vi "Control_stage_2.vi"(11 "Stage control":T3={"Up"=FALSE, "Left"=FALSE, "Right"=FALSE, "Down"=FALSE, "Z Down"=FALSE, "Z Up"=FALSE, "X Step Size(um)"=0.0, "Z step size (um)"=0.0, "Y Step Size(um)"=0.0, "Enable x-axis"=TRUE, "Enable y-axis"=TRUE, "Enable z-axis"=TRUE, "Same step size"=FALSE, "Global step size"=10.0, "stop"=FALSE, "Destination"={"X Position"=0.0, "Y Position"=0.0, "Z Position"=0.0}, "Move to destination"=FALSE}) -> (10 "Stage position":T2)   [LabVIEW 2020]
uses:
  typedefs/typedef_stage_control.ctl
  typedefs/typedef_stage_position.ctl
  typedefs/typedef_Z_stack.ctl
panel:
  in  "Z-stack":T1 {"Progress" scale=0.0..100.0}
  out "Error out":errorcluster
  out "Connected":bool=TRUE
  out "FirmwareVersion":string="3.03\r"
  in  "SPIIPLUSCOM660Lib.IAsyncChannel":refnum<k7>
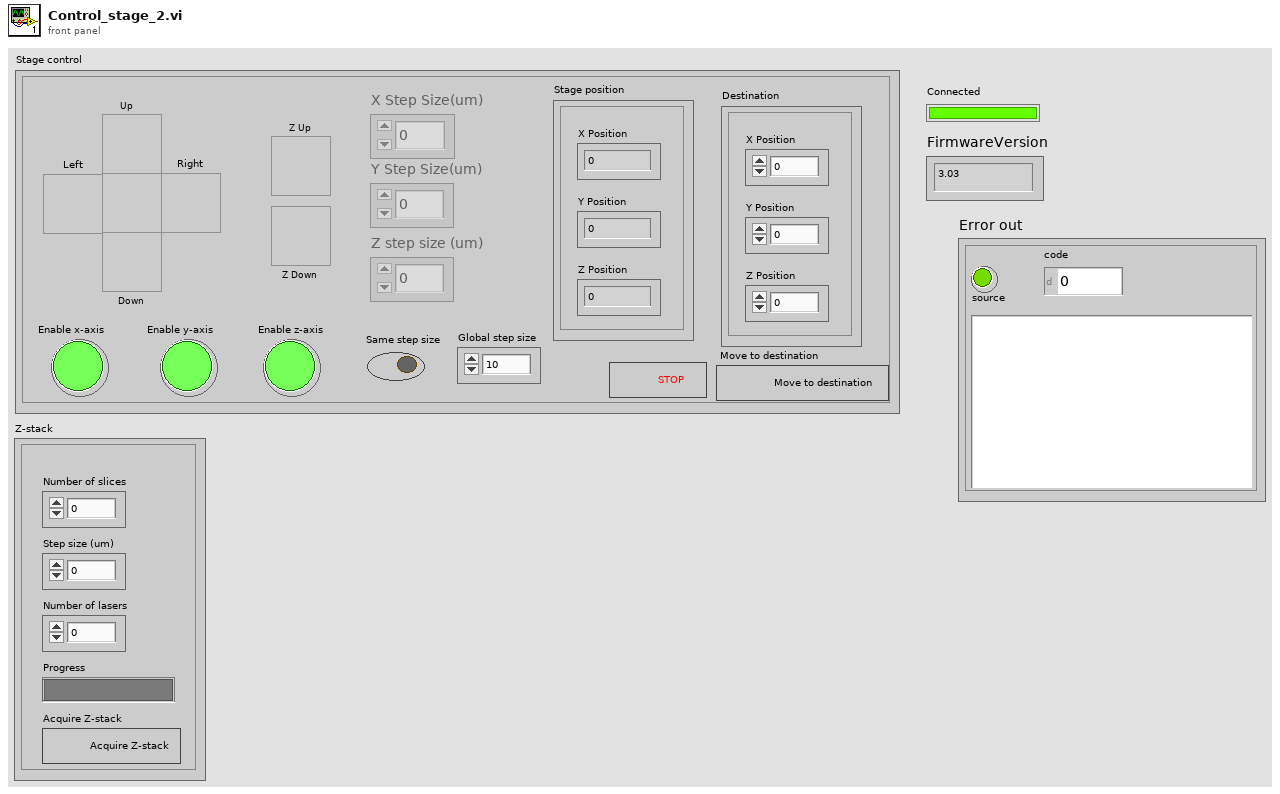
[diagram p1: front panel]
types:
  T1 = typedef "typedef_Z_stack.ctl" = cluster{"Acquire Z-stack":bool, "Step size (um)":dbl, "Number of slices":dbl, "Number of lasers":dbl, "Progress":u8}
  T2 = typedef "typedef_stage_position.ctl" = cluster{"X Position":dbl, "Y Position":dbl, "Z Position":dbl}
  T3 = typedef "typedef_stage_control.ctl" = cluster{"Up":bool, "Left":bool, "Right":bool, "Down":bool, "Z Down":bool, "Z Up":bool, "X Step Size(um)":dbl, "Z step size (um)":dbl, "Y Step Size(um)":dbl, "Enable x-axis":bool, "Enable y-axis":bool, "Enable z-axis":bool, "Same step size":bool, "Global step size":dbl, "stop":bool, "Destination":T2, "Move to destination":bool}
  T4 = enum16{"Initialize", "Verify connection", "Running", "Closing"}
  T5 = enum8{"Enabled", "Disabled", "Disabled and Grayed Out"}
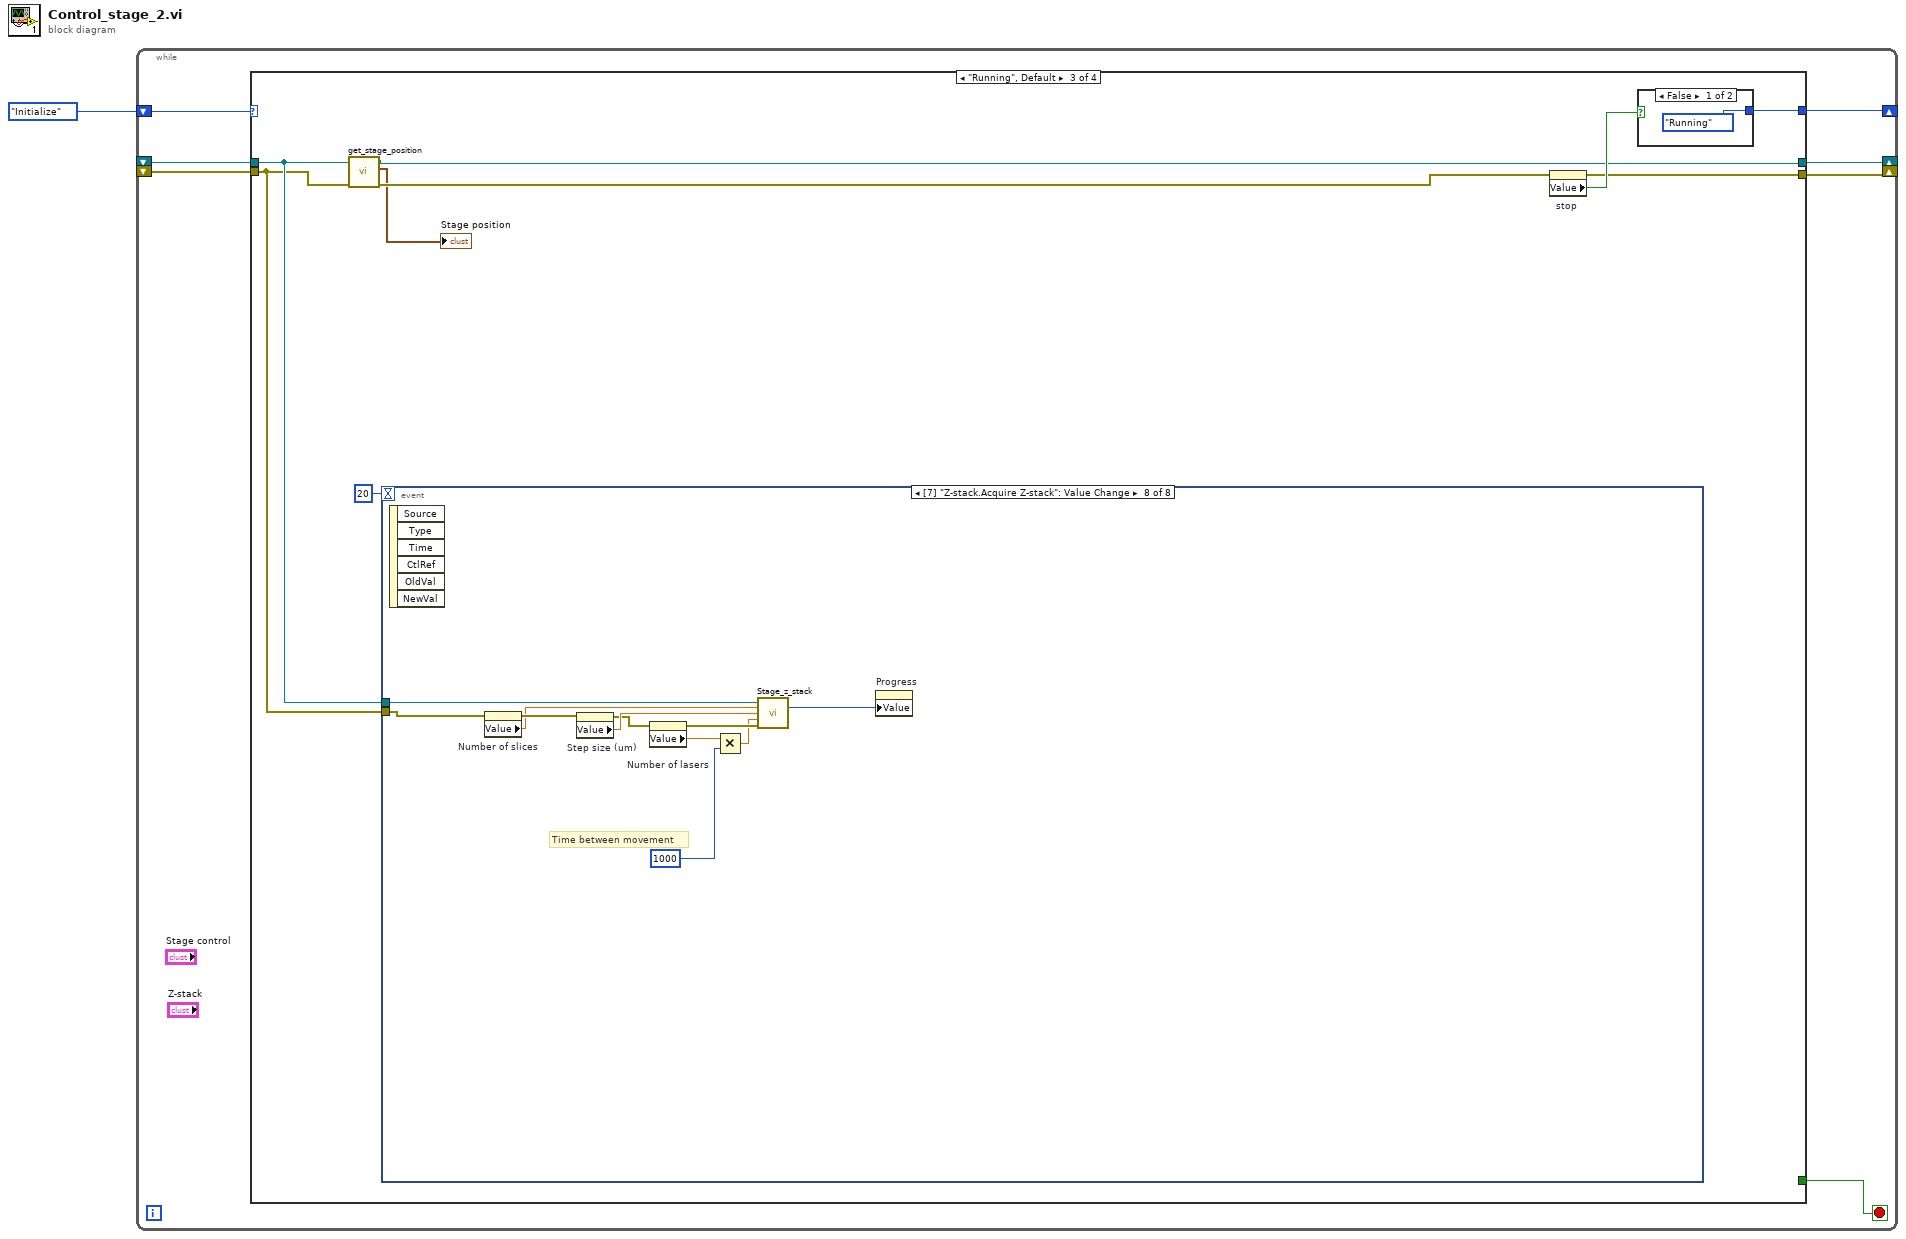
[diagram p0: block diagram]
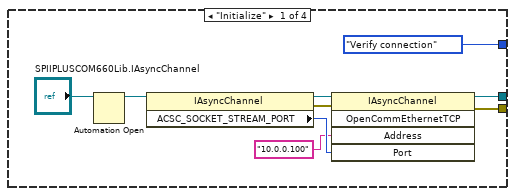
[diagram p2: hidden frame]
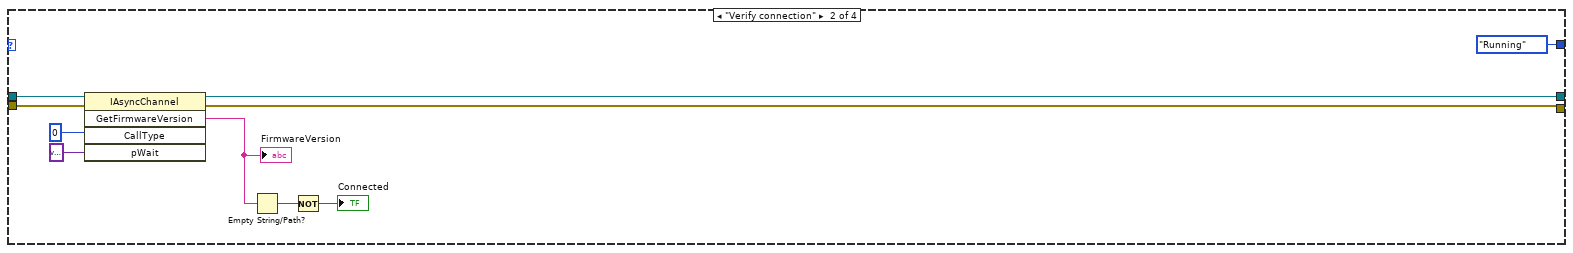
[diagram p3: hidden frame]
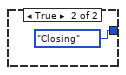
[diagram p4: hidden frame]
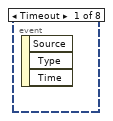
[diagram p5: hidden frame]
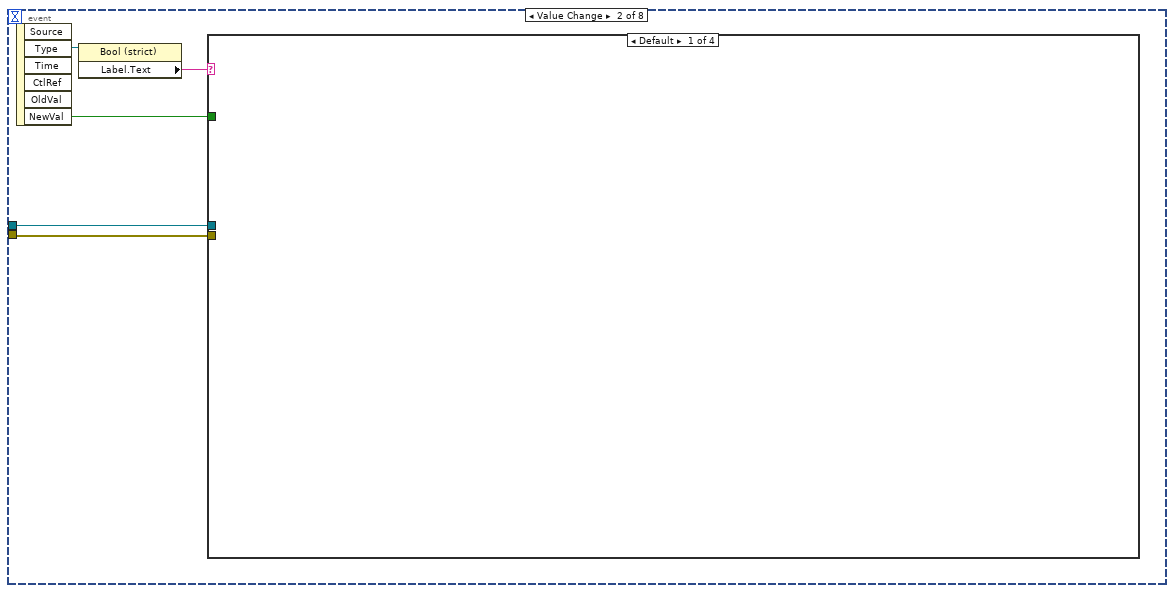
[diagram p6: hidden frame]
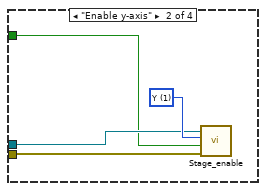
[diagram p7: hidden frame]
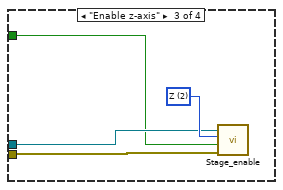
[diagram p8: hidden frame]
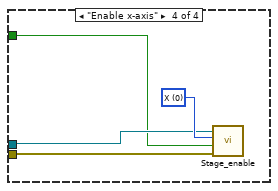
[diagram p9: hidden frame]
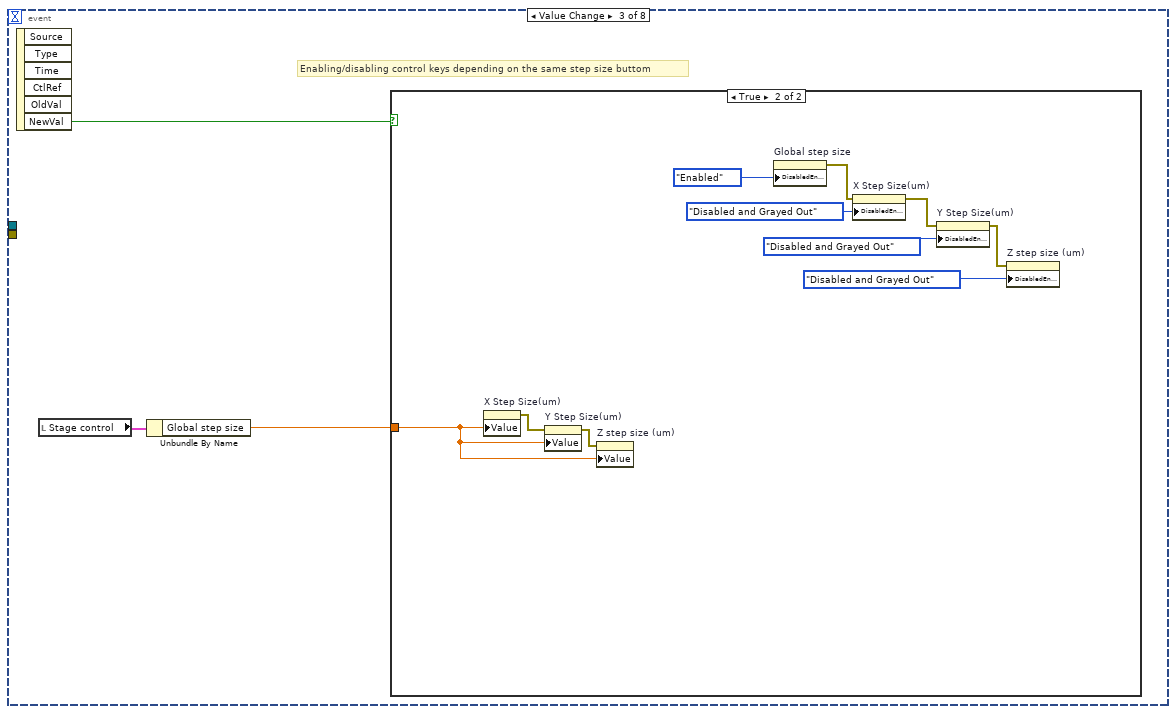
[diagram p10: hidden frame]
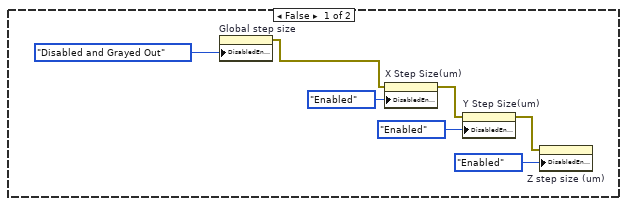
[diagram p11: hidden frame]
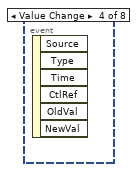
[diagram p12: hidden frame]
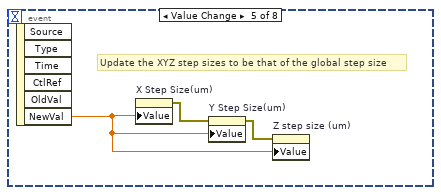
[diagram p13: hidden frame]
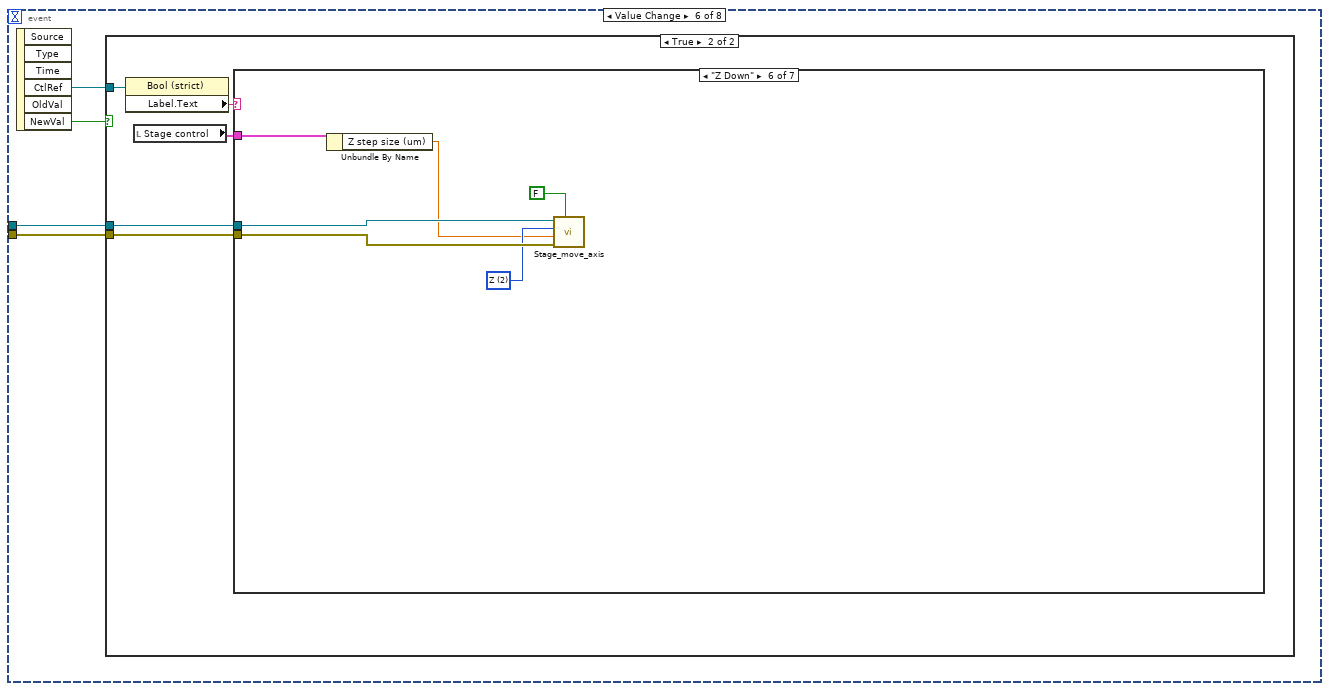
[diagram p14: hidden frame]
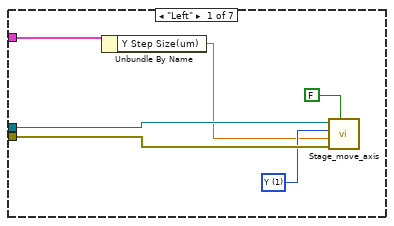
[diagram p16: hidden frame]
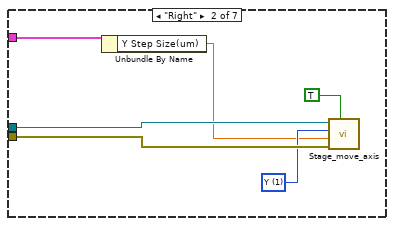
[diagram p17: hidden frame]
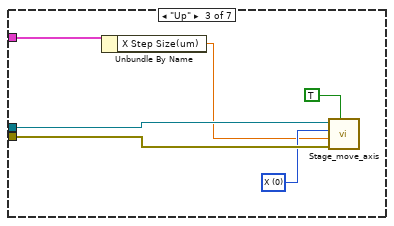
[diagram p18: hidden frame]
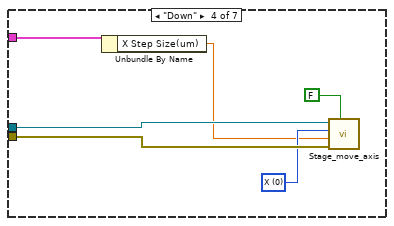
[diagram p19: hidden frame]
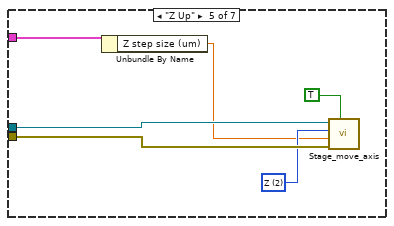
[diagram p20: hidden frame]
diagram:
  n1 = while {
    shift-right: [w4] -> _
    shift-left: T4."Initialize" -> [w7]
    shift-right: [w6] -> _
    shift-left: _ -> [w3]
    shift-right: [w5] -> _
    shift-left: _ -> [w2]
    stop <- w8 stop-if-true
    n2 = case shown="\"Running\", Default" w7 {
      tunnel: [_ _ _ TRUE ("NewVal")] -> w8
      tunnel: [w11 w20 w30 _] -> w6
      tunnel: [w10 w19 w34 _] -> w5
      tunnel: [T4."Verify connection" T4."Running" w36 _] -> w4
      tunnel: w3 -> [_ w22 w32 w163]
      tunnel: w2 -> [_ w21 w31 w162]
      frame "Initialize" {
        n3 = Automation Open(Automation Refnum="SPIIPLUSCOM660Lib.IAsyncChannel") -> (Automation Refnum=w17:refnum<k7>)  [unwired: 3 in, 1 out]
        n4 = property class="IAsyncChannel"(reference=w17) -> (reference out=w16:refnum<k7>, error out=w12:errorcluster, "ACSC_SOCKET_STREAM_PORT"=w14:i32)  [unwired: 1 in]
        n5 = invoke class="IAsyncChannel" method="OpenCommEthernetTCP"(reference=w16, error in=w12, "Address"="10.0.0.100", "Port"=w14) -> (reference out=w11:refnum<k7>, error out=w10:errorcluster)  [unwired: 1 in, 3 out]
      }
      frame "Verify connection" {
        n6 = invoke class="IAsyncChannel" method="GetFirmwareVersion"(reference=w22, error in=w21, "CallType"=u64 0, "pWait"=variant) -> (reference out=w20:refnum<k7>, error out=w19:errorcluster, "GetFirmwareVersion"=w25:string)  [unwired: 1 in, 2 out]
        "FirmwareVersion" <- w25
        n7 = Empty String/Path?(string/path=w25) -> (empty?=w24:bool)
        n8 = Not(x=w24) -> (.not. x?=→"Connected":bool)
      }
      frame "Running", Default {
        n9 = call "get_stage_position.vi"("error IN"=w31, "reference IN"=w32) -> ("error OUT"=w29:errorcluster, "Stage position OUT"=→"Stage position":T2, "reference OUT"=w30:refnum<k7>)  [unwired: 7 in]
        n10 = event shown="[7] \"Z-stack.Acquire Z-stack\": Value Change" {
          selector: _ -> [_ _ _ _ _ _ _ _]
          dyn-events: _ -> [_ _ _ _ _ _ _ _]
          timeout: 20 -> [_ _ _ _ _ _ _ _]
          tunnel: w32 -> [_ w40 _ _ _ w80 w149 w160]
          tunnel: w31 -> [_ w39 _ _ _ w79 w148 w159]
          event Timeout {
            n11 = event-data() -> ()  [unwired: 1 in, 3 out]
          }
          event Value Change {
            n12 = event-data() -> ("CtlRef"=w43:refnum<vi>, "NewVal"=w41:bool)  [unwired: 1 in, 4 out]
            n13 = property class="Bool (strict)"(reference=w43) -> ("Label.Text"=w42:string)  [unwired: 1 in, 2 out]
            n14 = case shown="Default" w42 {
              tunnel: w41 -> [_ w44 w48 w52]
              tunnel: w40 -> [_ w45 w50 w54]
              tunnel: w39 -> [_ w46 w49 w53]
              frame Default {
              }
              frame "Enable y-axis" {
                w47 = u16 1 items=["X", "Y", "Z"] ("Axes Select")
                n15 = call "Stage_enable.vi"("error in (no error)"=w46, "Boolean"=w44, "Axes Select"=w47, "reference"=w45) -> ()  [unwired: 6 in, 2 out]
              }
              frame "Enable z-axis" {
                w51 = u16 2 items=["X", "Y", "Z"] ("Axes Select")
                n16 = call "Stage_enable.vi"("error in (no error)"=w49, "Boolean"=w48, "Axes Select"=w51, "reference"=w50) -> ()  [unwired: 6 in, 2 out]
              }
              frame "Enable x-axis" {
                w55 = u16 0 items=["X", "Y", "Z"] ("Axes Select")
                n17 = call "Stage_enable.vi"("error in (no error)"=w53, "Boolean"=w52, "Axes Select"=w55, "reference"=w54) -> ()  [unwired: 6 in, 2 out]
              }
            }
          }
          event Value Change {
            # "Enabling/disabling control keys depending on the same step size buttom"
            n18 = event-data() -> ("NewVal"=w58:bool)  [unwired: 1 in, 5 out]
            n19 = local read "Stage control"() -> (w57:T3)
            n20 = Unbundle By Name(w57) -> ("Global step size"=w56:dbl)
            n21 = case shown="True" w58 {
              tunnel: w56 -> [_ w70]
              frame False {
                n22 = property on="Global step size" class="DigNum (strict)"("DisabledEnum"=T5."Disabled and Grayed Out" ("Disabled")) -> (error out=w59:errorcluster)  [unwired: 2 in, 1 out]
                n23 = property on="X Step Size(um)" class="DigNum (strict)"(error in=w59, "DisabledEnum"=T5."Enabled" ("Disabled")) -> (error out=w63:errorcluster)  [unwired: 1 in, 1 out]
                n24 = property on="Y Step Size(um)" class="DigNum (strict)"(error in=w63, "DisabledEnum"=T5."Enabled" ("Disabled")) -> (error out=w61:errorcluster)  [unwired: 1 in, 1 out]
                n25 = property on="Z step size (um)" class="DigNum (strict)"(error in=w61, "DisabledEnum"=T5."Enabled" ("Disabled")) -> ()  [unwired: 1 in, 2 out]
              }
              frame True {
                n26 = property on="X Step Size(um)" class="DigNum (strict)"("Value"=w70) -> (error out=w69:errorcluster)  [unwired: 2 in, 1 out]
                n27 = property on="Y Step Size(um)" class="DigNum (strict)"(error in=w69, "Value"=w70) -> (error out=w68:errorcluster)  [unwired: 1 in, 1 out]
                n28 = property on="Z step size (um)" class="DigNum (strict)"(error in=w68, "Value"=w70) -> ()  [unwired: 1 in, 2 out]
                n29 = property on="Global step size" class="DigNum (strict)"("DisabledEnum"=T5."Enabled" ("Disabled")) -> (error out=w66:errorcluster)  [unwired: 2 in, 1 out]
                n30 = property on="X Step Size(um)" class="DigNum (strict)"(error in=w66, "DisabledEnum"=T5."Disabled and Grayed Out" ("Disabled")) -> (error out=w73:errorcluster)  [unwired: 1 in, 1 out]
                n31 = property on="Y Step Size(um)" class="DigNum (strict)"(error in=w73, "DisabledEnum"=T5."Disabled and Grayed Out" ("Disabled")) -> (error out=w71:errorcluster)  [unwired: 1 in, 1 out]
                n32 = property on="Z step size (um)" class="DigNum (strict)"(error in=w71, "DisabledEnum"=T5."Disabled and Grayed Out" ("Disabled")) -> ()  [unwired: 1 in, 2 out]
              }
            }
          }
          event Value Change {
            n33 = event-data() -> ()  [unwired: 1 in, 6 out]
          }
          event Value Change {
            # "Update the XYZ step sizes to be that of the global step size"
            n34 = event-data() -> ("NewVal"=w78:dbl)  [unwired: 1 in, 5 out]
            n35 = property on="X Step Size(um)" class="DigNum (strict)"("Value"=w78) -> (error out=w77:errorcluster)  [unwired: 2 in, 1 out]
            n36 = property on="Y Step Size(um)" class="DigNum (strict)"(error in=w77, "Value"=w78) -> (error out=w76:errorcluster)  [unwired: 1 in, 1 out]
            n37 = property on="Z step size (um)" class="DigNum (strict)"(error in=w76, "Value"=w78) -> ()  [unwired: 1 in, 2 out]
          }
          event Value Change {
            n38 = event-data() -> ("CtlRef"=w82:refnum<vi>, "NewVal"=w81:bool)  [unwired: 1 in, 4 out]
            n39 = case shown="True" w81 {
              tunnel: w82 -> [_ w87]
              tunnel: w80 -> [_ w84]
              tunnel: w79 -> [_ w83]
              frame False {
              }
              frame True {
                n40 = property class="Bool (strict)"(reference=w87) -> ("Label.Text"=w86:string)  [unwired: 1 in, 2 out]
                n41 = local read "Stage control"() -> (w85:T3)
                n42 = case shown="\"Z Down\"" w86 {
                  tunnel: w85 -> [w93 w99 w105 w111 w117 w123 _]
                  tunnel: w84 -> [w92 w98 w104 w110 w116 w122 _]
                  tunnel: w83 -> [w91 w97 w103 w109 w115 w121 _]
                  frame "Left" {
                    w89 = u16 1 items=["X", "Y", "Z"] ("Axes Select")
                    n43 = Unbundle By Name(w93) -> ("Y Step Size(um)"=w88:dbl)
                    n44 = call "Stage_move_axis.vi"("Direction true means positive increment"=FALSE, "error in (no error)"=w91, "Distance micrometer"=w88, "Axes Select"=w89, "reference IN"=w92) -> ()  [unwired: 5 in, 2 out]
                  }
                  frame "Right" {
                    w95 = u16 1 items=["X", "Y", "Z"] ("Axes Select")
                    n45 = Unbundle By Name(w99) -> ("Y Step Size(um)"=w94:dbl)
                    n46 = call "Stage_move_axis.vi"("Direction true means positive increment"=TRUE, "error in (no error)"=w97, "Distance micrometer"=w94, "Axes Select"=w95, "reference IN"=w98) -> ()  [unwired: 5 in, 2 out]
                  }
                  frame "Up" {
                    w101 = u16 0 items=["X", "Y", "Z"] ("Axes Select")
                    n47 = Unbundle By Name(w105) -> ("X Step Size(um)"=w100:dbl)
                    n48 = call "Stage_move_axis.vi"("Direction true means positive increment"=TRUE, "error in (no error)"=w103, "Distance micrometer"=w100, "Axes Select"=w101, "reference IN"=w104) -> ()  [unwired: 5 in, 2 out]
                  }
                  frame "Down" {
                    w107 = u16 0 items=["X", "Y", "Z"] ("Axes Select")
                    n49 = Unbundle By Name(w111) -> ("X Step Size(um)"=w106:dbl)
                    n50 = call "Stage_move_axis.vi"("Direction true means positive increment"=FALSE, "error in (no error)"=w109, "Distance micrometer"=w106, "Axes Select"=w107, "reference IN"=w110) -> ()  [unwired: 5 in, 2 out]
                  }
                  frame "Z Up" {
                    w113 = u16 2 items=["X", "Y", "Z"] ("Axes Select")
                    n51 = Unbundle By Name(w117) -> ("Z step size (um)"=w112:dbl)
                    n52 = call "Stage_move_axis.vi"("Direction true means positive increment"=TRUE, "error in (no error)"=w115, "Distance micrometer"=w112, "Axes Select"=w113, "reference IN"=w116) -> ()  [unwired: 5 in, 2 out]
                  }
                  frame "Z Down" {
                    w119 = u16 2 items=["X", "Y", "Z"] ("Axes Select")
                    n53 = Unbundle By Name(w123) -> ("Z step size (um)"=w118:dbl)
                    n54 = call "Stage_move_axis.vi"("Direction true means positive increment"=FALSE, "error in (no error)"=w121, "Distance micrometer"=w118, "Axes Select"=w119, "reference IN"=w122) -> ()  [unwired: 5 in, 2 out]
                  }
                  frame Default {
                  }
                }
              }
            }
          }
          event Value Change {
            w138 = u16 2 items=["X", "Y", "Z"] ("Axes Select")
            w142 = u16 1 items=["X", "Y", "Z"] ("Axes Select")
            w144 = u16 0 items=["X", "Y", "Z"] ("Axes Select")
            n55 = event-data() -> ()  [unwired: 1 in, 6 out]
            n56 = call "get_stage_position.vi"("error IN"=w148, "reference IN"=w149) -> ("error OUT"=w146:errorcluster, "Stage position OUT"=w131:T2, "reference OUT"=w147:refnum<k7>)  [unwired: 7 in]
            n57 = property on="Destination" class="Clust (strict)"(error in=w146) -> (error out=w145:errorcluster, "Value"=w132:T2)  [unwired: 1 in, 1 out]
            n58 = Subtract(x=w131, y=w132) -> (x-y=w129:T2)
            n59 = Multiply(x=w129, y=T2 {"X Position"=1000.0, "Y Position"=1000.0, "Z Position"=1000.0}) -> (x*y=w127:T2)
            n60 = Unbundle By Name(w127) -> ("X Position"=w143:dbl, "Y Position"=w139:dbl, "Z Position"=w130:dbl)
            n61 = call "Stage_move_axis.vi"("Direction true means positive increment"=FALSE, "error in (no error)"=w145, "Distance micrometer"=w143, "Axes Select"=w144, "reference IN"=w147) -> ("error OUT"=w140:errorcluster, "reference OUT"=w141:refnum<k7>)  [unwired: 5 in]
            n62 = call "Stage_move_axis.vi"("Direction true means positive increment"=FALSE, "error in (no error)"=w140, "Distance micrometer"=w139, "Axes Select"=w142, "reference IN"=w141) -> ("error OUT"=w137:errorcluster, "reference OUT"=w136:refnum<k7>)  [unwired: 5 in]
            n63 = call "Stage_move_axis.vi"("Direction true means positive increment"=FALSE, "error in (no error)"=w137, "Distance micrometer"=w130, "Axes Select"=w138, "reference IN"=w136) -> ("error OUT"=w134:errorcluster, "reference OUT"=w135:refnum<k7>)  [unwired: 5 in]
            n64 = call "get_stage_position.vi"("error IN"=w134, "reference IN"=w135) -> ("Stage position OUT"=w133:T2)  [unwired: 7 in, 2 out]
            n65 = local write "Stage position"(w133) -> ()
          }
          event Value Change {
            # "Time between movement"
            n66 = event-data() -> ()  [unwired: 1 in, 6 out]
            n67 = property on="Number of slices" class="DigNum (strict)"(error in=w159) -> (error out=w158:errorcluster, "Value"=w150:dbl)  [unwired: 1 in, 1 out]
            n68 = property on="Step size (um)" class="DigNum (strict)"(error in=w158) -> (error out=w156:errorcluster, "Value"=w157:dbl)  [unwired: 1 in, 1 out]
            n69 = property on="Number of lasers" class="DigNum (strict)"(error in=w156) -> (error out=w155:errorcluster, "Value"=w153:dbl)  [unwired: 1 in, 1 out]
            n70 = Multiply(x=w153, y=1000) -> (x*y=w152:dbl)
            n71 = call "Stage_z_stack.vi"("SPIIPLUSCOM660Lib.IAsyncChannel IN"=w160, "Number of slices"=w150, "Z step size (um)"=w157, "delay between steps (ms)"=w152, "error IN"=w155) -> ("Progress bar"=w151:u8)  [unwired: 7 in, 3 out]
            n72 = property on="Progress" class="Slide (strict)"("Value"=w151) -> ()  [unwired: 2 in, 2 out]
          }
        }
        n73 = property on="stop" class="Bool (strict)"(error in=w29) -> (error out=w34:errorcluster, "Value"=w35:bool)  [unwired: 1 in, 1 out]
        n74 = case shown="False" w35 {
          tunnel: [T4."Running" T4."Closing"] -> w36
          frame False {
          }
          frame True {
          }
        }
      }
      frame "Closing" {
        n75 = local write "Connected"(FALSE ("Connected")) -> ()
        n76 = invoke class="IAsyncChannel" method="CloseComm"(reference=w163, error in=w162) -> (error out=→"Error out":errorcluster)  [unwired: 1 in, 2 out]
      }
    }
  }
